vi "get_saved_pos_array.vi"(8 "error in (no error)":errorcluster caption="错误输入（无错误）", 11 "MotorSystem输入":refnum<class "MotorSystem.lvclass">) -> (0 "error out":errorcluster caption="错误输出", 2 "saved pos array":T1[](array[typedef]), 3 "MotorSystem输出":refnum<class "MotorSystem.lvclass">)   [LabVIEW 2016, in "MotionControl.lvlib" / "MotorSystem.lvclass"]
uses:
  <userlib>/MotionControl/MotorSystem/MotorSystem.lvclass
  <userlib>/MotionControl/MotorSystem/SavedPosCluster.ctl
  <userlib>/MotionControl/MotorSystem/CommandList.ctl
  <userlib>/MotionControl/MotorSystem/cmd_system.ctl
  <userlib>/MotionControl/MotorSystem/SavedDimensionCluster.ctl
  <userlib>/MotionControl/OneMotion/unit mode.ctl
  <userlib>/MotionControl/MotorSystem/MotorSystem.lvclass/MotorSystem.ctl
  <userlib>/MotionControl/OneMotion/OneMotion.lvclass
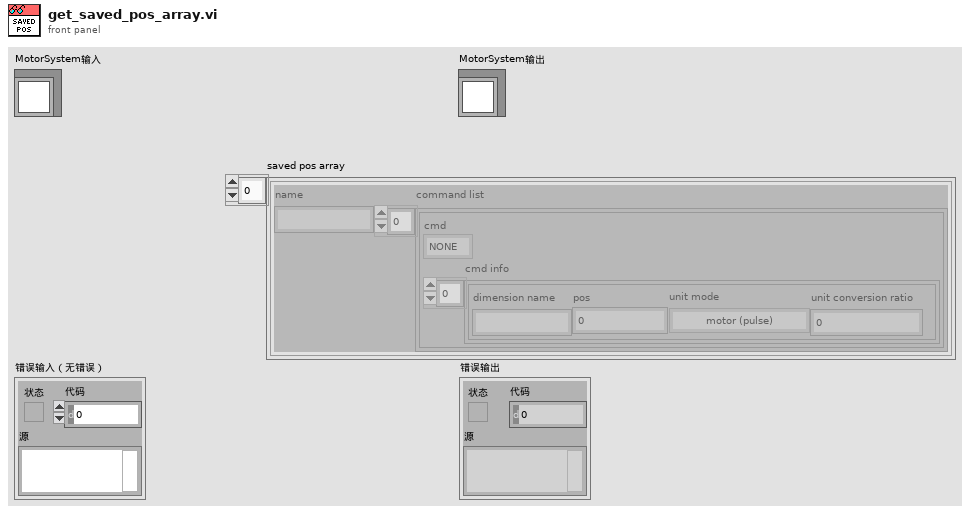
[diagram p1: front panel]
types:
  T1 = typedef "MotionControl.lvlib/MotorSystem.lvclass/SavedPosCluster.ctl" = cluster{"name":string, "command list":T2}
  T2 = typedef "MotionControl.lvlib/MotorSystem.lvclass/CommandList.ctl" = cluster{"cmd":T3, "cmd info":T4[]}[]
  T3 = typedef "MotionControl.lvlib/MotorSystem.lvclass/cmd_system.ctl" = enum16{"NONE", "MOVE_SYSTEM", "WAIT_UNTIL_MOVE_DONE", "EXIT"}
  T4 = typedef "MotionControl.lvlib/MotorSystem.lvclass/SavedDimensionCluster.ctl" = cluster{"dimension name":string, "pos":dbl, "unit mode":T5, "unit conversion ratio":dbl}
  T5 = typedef "MotionControl.lvlib/OneMotion.lvclass/unit mode.ctl" = enum16{"motor (pulse)", "linear (mm) or radial (degree)"}
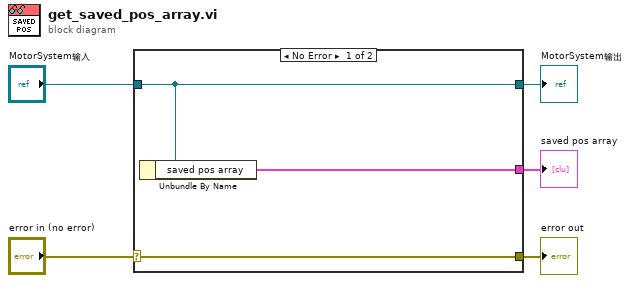
[diagram p0: block diagram]
diagram:
  n1 = case shown="No Error" "error in (no error)" {
    selector: "error in (no error)" -> [w8 w9]
    tunnel: [w8 w9] -> w4
    tunnel: [w7 w10] -> w2
    tunnel: "MotorSystem输入" -> [w7 w10]
    tunnel: [w6 _] -> w1
    frame No Error {
      n2 = Unbundle By Name(w7) -> ("saved pos array"=w6:T1[])
    }
    frame Error {
    }
  }
  "error out" <- w4
  "MotorSystem输出" <- w2
  "saved pos array" <- w1
